vi "Local Variable.vi"() -> ()   [LabVIEW 2015]
panel:
  out "Numeric 2":dbl
  out "Numeric":dbl
  in  "Boolean":bool
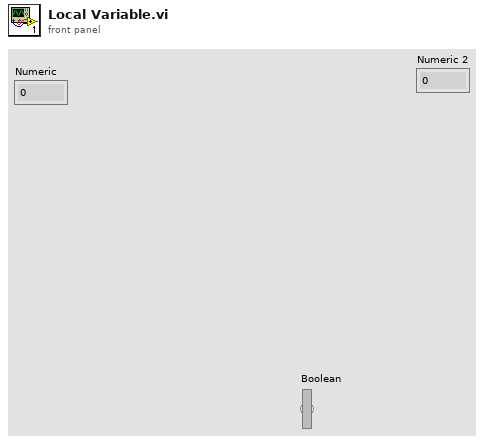
[diagram p1: front panel]
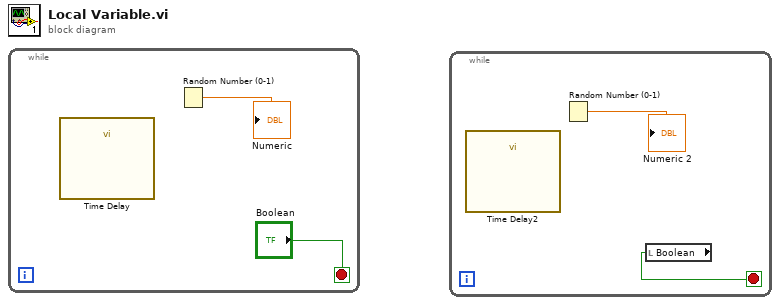
[diagram p0: block diagram]
diagram:
  n1 = while {
    stop <- "Boolean" stop-if-true
    n2 = call "Time Delay"() -> ()  [unwired: 11 in, 1 out]
    n3 = Random Number (0-1)() -> (number: 0 to 1=→"Numeric":dbl)
  }
  n4 = while {
    stop <- w4 stop-if-true
    n5 = call "Time Delay2"() -> ()  [unwired: 11 in, 1 out]
    n6 = Random Number (0-1)() -> (number: 0 to 1=→"Numeric 2":dbl)
    n7 = local read "Boolean"() -> (w4:bool)
  }
